vi "TCP_ESP32_excel.vi"() -> ()   [LabVIEW 2021]
panel:
  out "Waveform Chart Crash Type":dbl[](graph)
  out "Waveform Chart Pitch":dbl[](graph)
  out "Waveform Chart A_z":dbl[](graph)
  out "Waveform Chart A_y":dbl[](graph)
  out "Waverform chart A_x":dbl[](graph)
  in  "stop":bool
  out "Waveform Chart Roll":dbl[](graph)
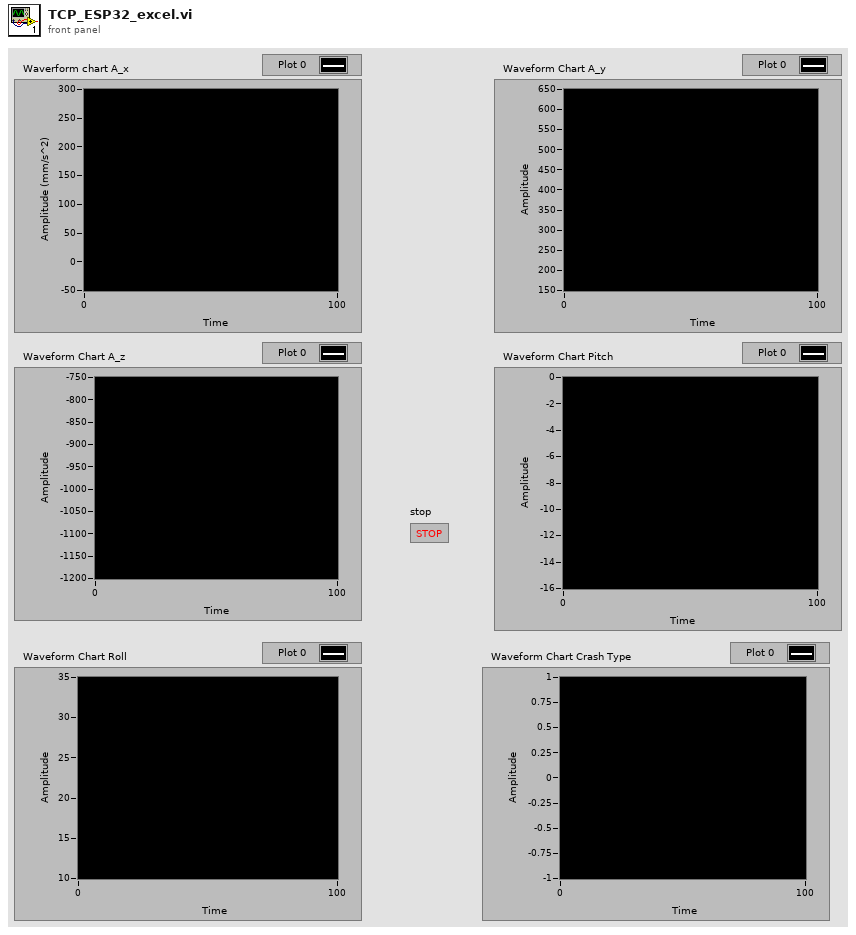
[diagram p1: front panel]
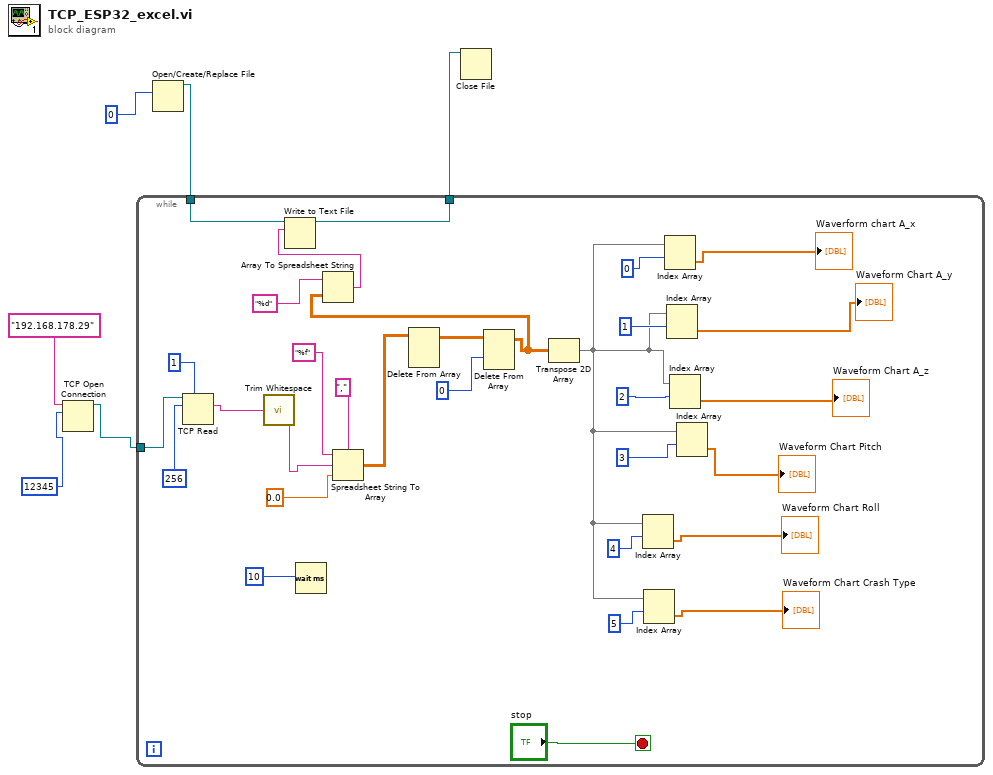
[diagram p0: block diagram]
diagram:
  n1 = TCP Open Connection(address="192.168.178.29", remote port or service name=12345) -> (connection ID=w4:refnum<k5>)  [unwired: 3 in, 1 out]
  n2 = Open/Create/Replace File(operation (0:open)=0) -> (refnum out=w2:refnum<file>)  [unwired: 5 in, 2 out]
  n3 = while {
    tunnel: w4 -> [w37]
    tunnel: w2 -> [w17]
    tunnel: [w16] -> w1
    stop <- "stop" stop-if-true
    n4 = TCP Read(connection ID=w37, bytes to read=256, 7:1) -> (data out=w36:string)  [unwired: 2 in, 2 out]
    n5 = call <vilib>:"Trim Whitespace.vi"("string"=w36) -> ("trimmed string"=w35:string)  [unwired: 1 in]
    n6 = Wait (ms)(milliseconds to wait=10) -> ()  [unwired: 1 out]
    n7 = Spreadsheet String To Array(delimiter (Tab)=",", format string="%f", spreadsheet string=w35, array type (2D Dbl)=0.0) -> (array=w24:dbl[][])
    n8 = Delete From Array(array=w24) -> (array with subset deleted=w28:dbl[][])  [unwired: 3 in, 1 out]
    n9 = Delete From Array(array=w28, index (row)=0) -> (array with subset deleted=w14:dbl[][])  [unwired: 2 in, 1 out]
    n10 = Array To Spreadsheet String(array=w14, 3:"%d") -> (spreadsheet string=w13:string)  [unwired: 1 in]
    n11 = Write to Text File(file (use dialog)=w17, text=w13) -> (refnum out=w16:refnum<file>)  [unwired: 2 in, 2 out]
    n12 = Transpose 2D Array(2D array=w14) -> (transposed array=w15:dbl[][])
    n13 = Index Array(array=w15, index (row)=4) -> (element=→"Waveform Chart Roll":dbl[])  [unwired: 1 in]
    n14 = Index Array(array=w15, index (row)=5) -> (element=→"Waveform Chart Crash Type":dbl[])  [unwired: 1 in]
    n15 = Index Array(array=w15, index (row)=0) -> (element=→"Waverform chart A_x":dbl[])  [unwired: 1 in]
    n16 = Index Array(array=w15, index (row)=1) -> (element=→"Waveform Chart A_y":dbl[])  [unwired: 1 in]
    n17 = Index Array(array=w15, index (row)=2) -> (element=→"Waveform Chart A_z":dbl[])  [unwired: 1 in]
    n18 = Index Array(array=w15, index (row)=3) -> (element=→"Waveform Chart Pitch":dbl[])  [unwired: 1 in]
  }
  n19 = Close File(refnum=w1) -> ()  [unwired: 1 in, 2 out]
